vi "DAQ-AI Mean Value.vi"(11 "data":dbl[][](array[numeric]) format="%0.2f") -> (3 "Analoge Input":dbl[](array[numeric]))   [LabVIEW 2015]
uses:
  <vilib>/Analysis/baseanly.llb/Mean (DBL).vi
  Galobal variable_TI.vi
  <vilib>/Analysis/NI_AALBase.lvlib
  <vilib>/ptbypt/NI_PtbyPt.lvlib
panel:
  out "Sensor Data":T1
  out "AI_as DI":bool[](array[boolean])
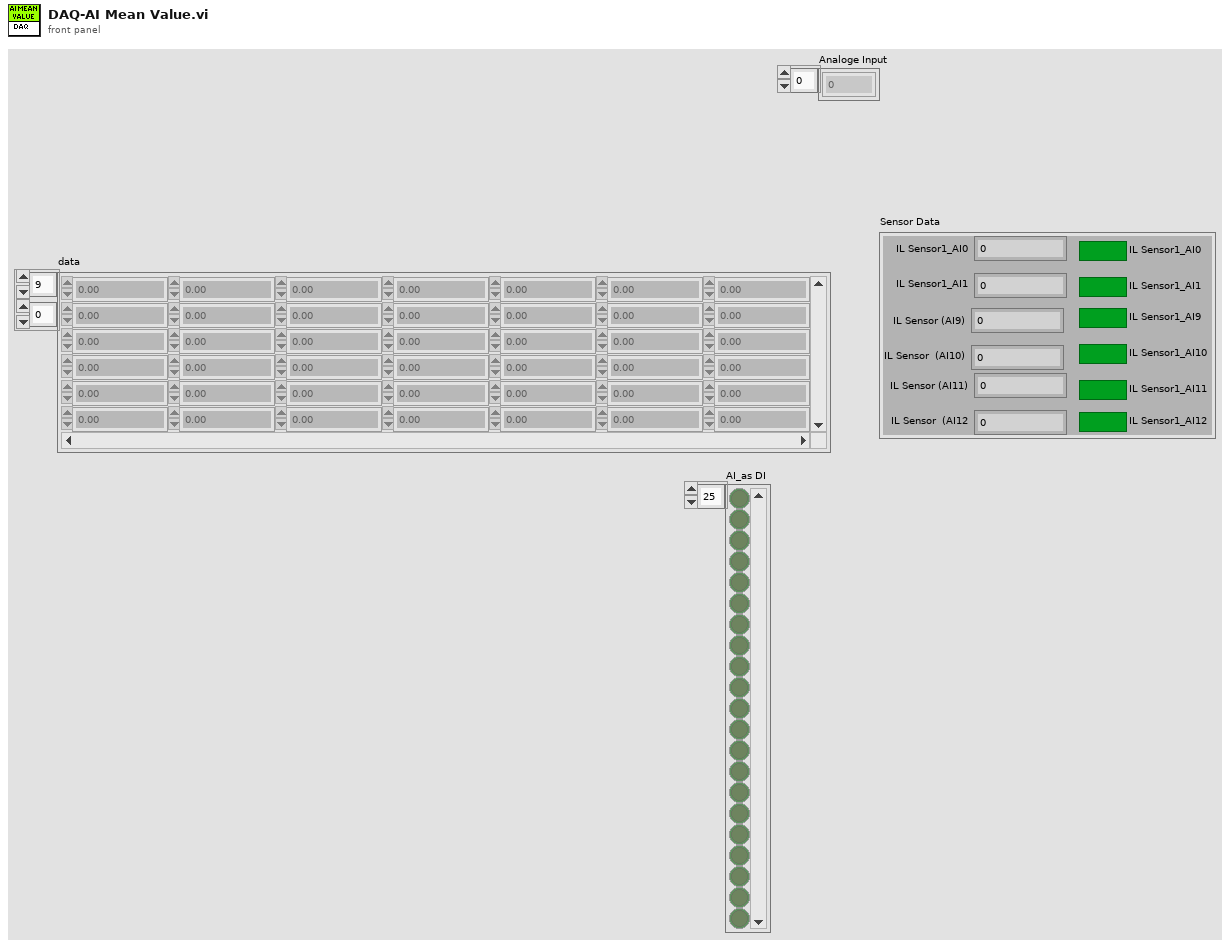
[diagram p1: front panel]
types:
  T1 = cluster{"IL Sensor1_AI0":dbl, "IL Sensor1_AI1":dbl, "IL Sensor (AI9)":dbl, "IL Sensor  (AI10)":dbl, "IL Sensor (AI11)":dbl, "IL Sensor  (AI12":dbl, "IL Sensor1_AI0":bool, "IL Sensor1_AI1":bool, "IL Sensor1_AI9":bool, "IL Sensor1_AI10":bool, "IL Sensor1_AI11":bool, "IL Sensor1_AI12":bool}
  T2 = cluster{"IL Sensor1_AI0":dbl, "IL Sensor1_AI1":dbl, "IL Sensor (AI6)":dbl, "IL Sensor  (AI7)":dbl, "IL Sensor (AI8)":dbl, "IL Sensor  (AI9)":dbl, "IL Sensor1_AI0":bool, "IL Sensor1_AI1":bool, "IL Sensor1_AI9":bool, "IL Sensor1_AI10":bool, "IL Sensor1_AI11":bool, "IL Sensor1_AI12":bool}
  T3 = cluster{"IL Sensor1_Max AI0":dbl, "IL Sensor1_Min AI0":dbl, "IL Sensor1_Max AI1":dbl, "IL Sensor1_ Min AI1":dbl, "IL Sensor_Max (AI9)":dbl, "IL Sensor_Min  (AI9)":dbl, "IL Sensor_Max (AI10)":dbl, "IL Sensor_Min(AI10)":dbl, "IL Sensor_Max (AI11)":dbl, "IL Sensor_Min (AI11)":dbl, "IL Sensor_Max (AI12)":dbl, "IL Sensor_Min (AI12":dbl}
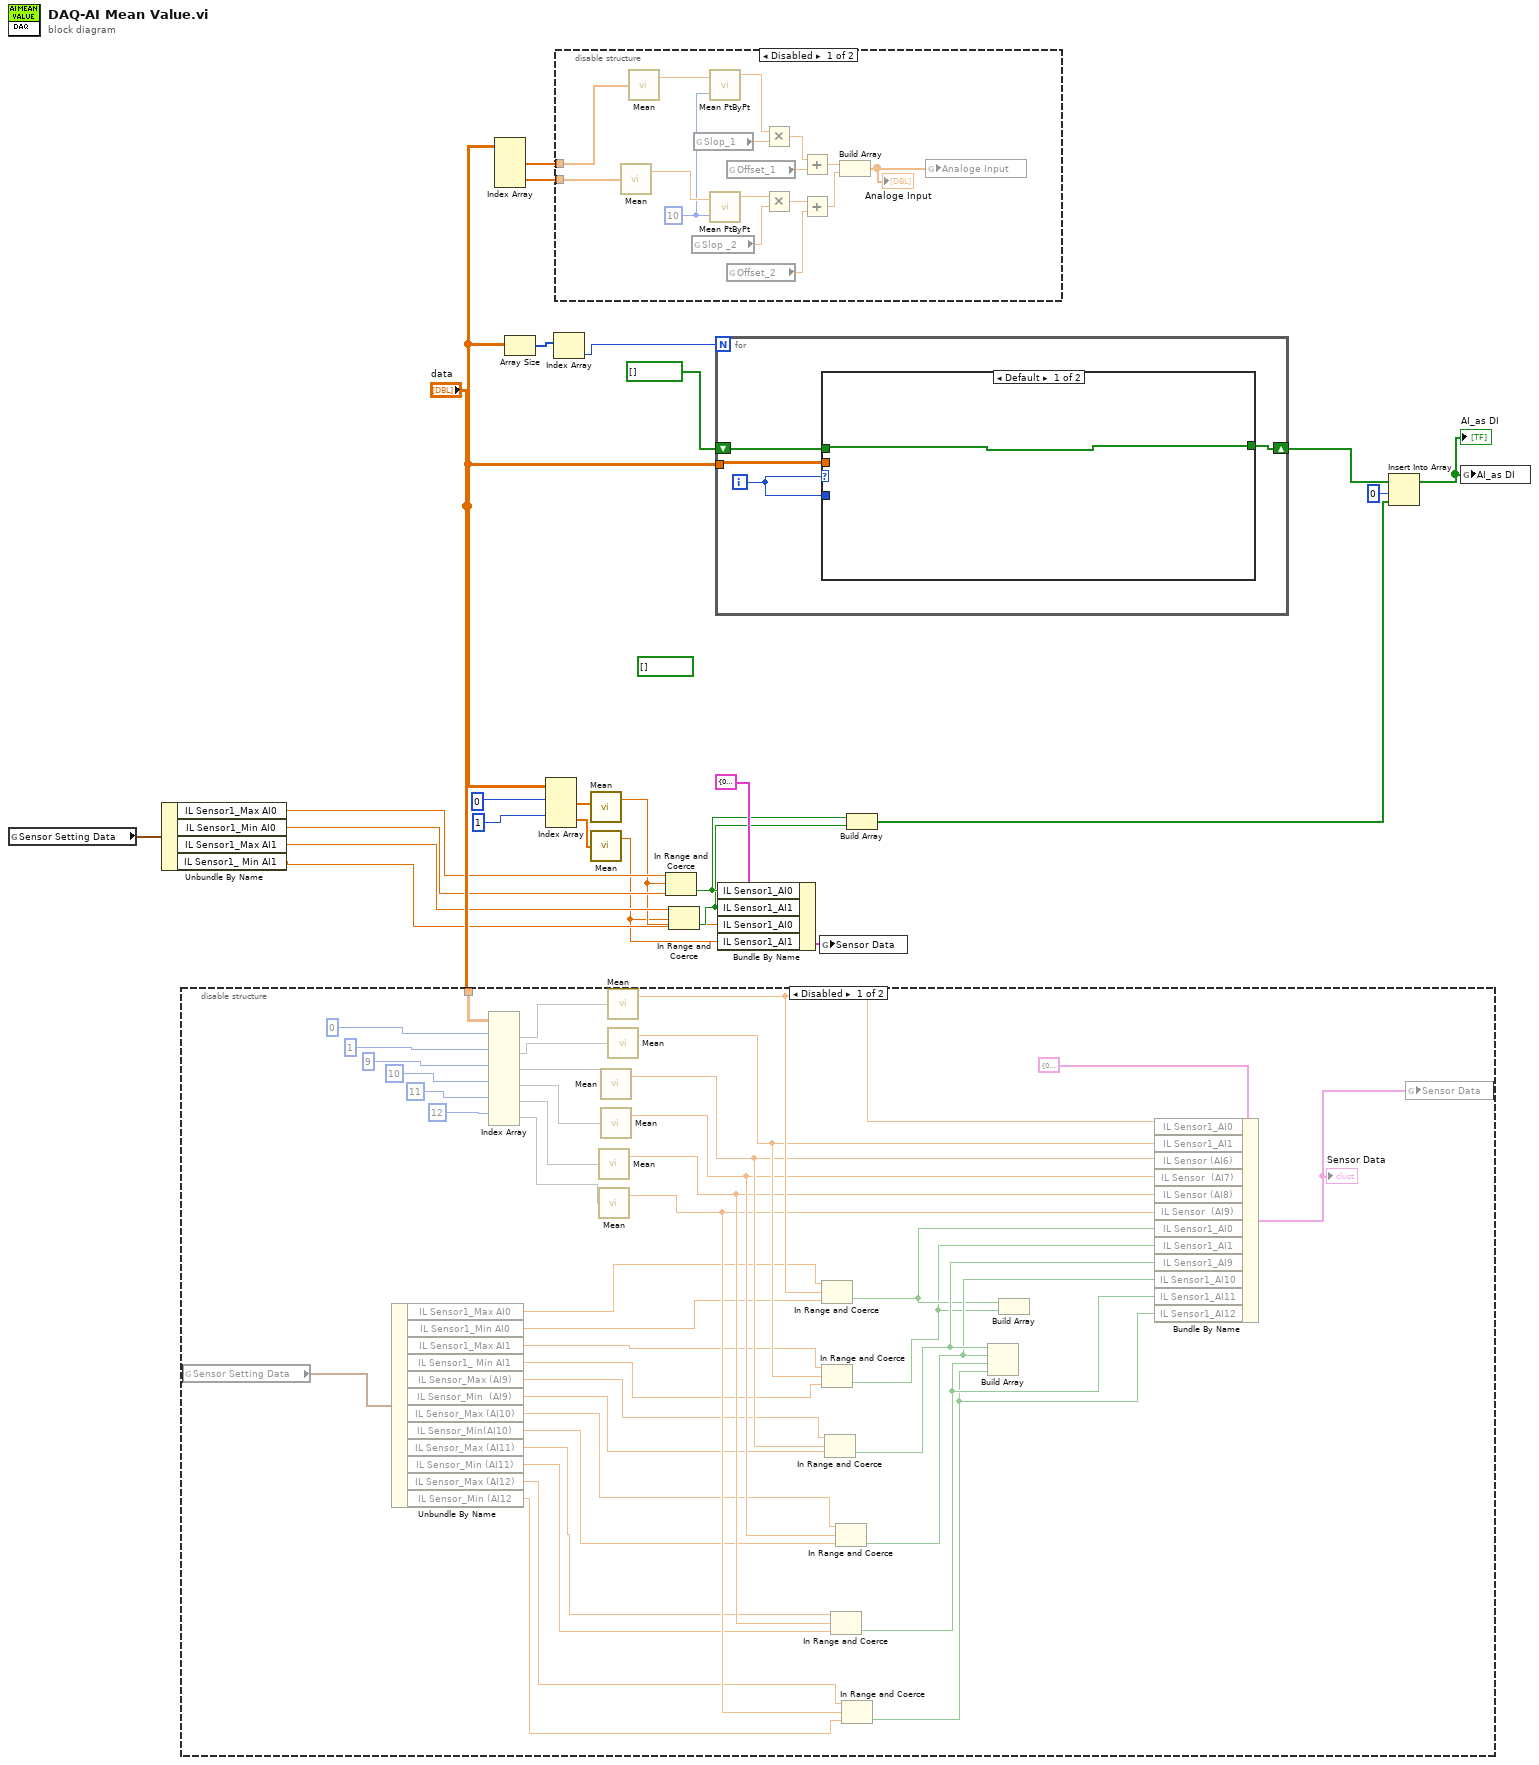
[diagram p0: block diagram]
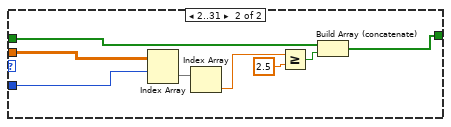
[diagram p4: hidden frame]
diagram:
  (unwired) bool[] []
  n1 = global read "Galobal variable_TI.vi" "Sensor Setting Data"() -> (w15:T3)
  n2 = Unbundle By Name(w15) -> ("IL Sensor1_Max AI0"=w14:dbl, "IL Sensor1_Min AI0"=w13:dbl, "IL Sensor1_Max AI1"=w12:dbl, "IL Sensor1_ Min AI1"=w11:dbl)
  n3 = disable-structure shown="Disabled" {
    disable-tunnel: "data" -> [w63 _]
    frame Disabled {
      n4 = global read "Galobal variable_TI.vi" "Sensor Setting Data"() -> (w26:T3)
      n5 = Unbundle By Name(w26) -> ("IL Sensor1_Max AI0"=w38:dbl, "IL Sensor1_Min AI0"=w37:dbl, "IL Sensor1_Max AI1"=w36:dbl, "IL Sensor1_ Min AI1"=w35:dbl, "IL Sensor_Max (AI9)"=w34:dbl, "IL Sensor_Min  (AI9)"=w33:dbl, "IL Sensor_Max (AI10)"=w32:dbl, "IL Sensor_Min(AI10)"=w31:dbl, "IL Sensor_Max (AI11)"=w30:dbl, "IL Sensor_Min (AI11)"=w29:dbl, "IL Sensor_Max (AI12)"=w28:dbl, "IL Sensor_Min (AI12"=w27:dbl)
      n6 = Index Array(array=w63, index (row) #1=0 ("index (row)"), index (row) #2=1 ("index (row)"), index (row) #3=9 ("index (row)"), index (row) #4=10 ("index (row)"), index (row) #5=11 ("index (row)"), index (row) #6=12 ("index (row)")) -> (element #1=w65:dbl[], element #2=w64:dbl[], element #3=w60:dbl[], element #4=w59:dbl[], element #5=w58:dbl[], element #6=w57:dbl[])  [unwired: 6 in]
      n7 = call-poly <vilib>:"Mean.vi"("X"=w58) -> ("mean"=w52:dbl)  [unwired: 1 out]
      n8 = call-poly <vilib>:"Mean.vi"("X"=w57) -> ("mean"=w51:dbl)  [unwired: 1 out]
      n9 = call-poly <vilib>:"Mean.vi"("X"=w60) -> ("mean"=w54:dbl)  [unwired: 1 out]
      n10 = call-poly <vilib>:"Mean.vi"("X"=w59) -> ("mean"=w53:dbl)  [unwired: 1 out]
      n11 = call-poly <vilib>:"Mean.vi"("X"=w65) -> ("mean"=w56:dbl)  [unwired: 1 out]
      n12 = call-poly <vilib>:"Mean.vi"("X"=w64) -> ("mean"=w55:dbl)  [unwired: 1 out]
      n13 = In Range and Coerce(upper limit=w38, x=w56, lower limit=w37) -> (In Range?=w49:bool)  [unwired: 1 out]
      n14 = In Range and Coerce(upper limit=w36, x=w55, lower limit=w35) -> (In Range?=w48:bool)  [unwired: 1 out]
      n15 = In Range and Coerce(upper limit=w34, x=w54, lower limit=w33) -> (In Range?=w62:bool)  [unwired: 1 out]
      n16 = In Range and Coerce(upper limit=w30, x=w52, lower limit=w29) -> (In Range?=w47:bool)  [unwired: 1 out]
      n17 = In Range and Coerce(upper limit=w32, x=w53, lower limit=w31) -> (In Range?=w61:bool)  [unwired: 1 out]
      n18 = In Range and Coerce(upper limit=w28, x=w51, lower limit=w27) -> (In Range?=w46:bool)  [unwired: 1 out]
      n19 = Build Array(w62, w61, w47, w46) -> ()  [unwired: 1 out]
      n20 = Build Array(w49, w48) -> ()  [unwired: 1 out]
      n21 = Bundle By Name(cluster=T2 {"IL Sensor1_AI0"=0.0, "IL Sensor1_AI1"=0.0, "IL Sensor (AI6)"=0.0, "IL Sensor  (AI7)"=0.0, "IL Sensor (AI8)"=0.0, "IL Sensor  (AI9)"=0.0, "IL Sensor1_AI0"=FALSE, "IL Sensor1_AI1"=FALSE, "IL Sensor1_AI9"=FALSE, "IL Sensor1_AI10"=FALSE, "IL Sensor1_AI11"=FALSE, "IL Sensor1_AI12"=FALSE} ("Sensor Data"), "IL Sensor1_AI0"=w56, "IL Sensor1_AI1"=w55, "IL Sensor (AI6)"=w54, "IL Sensor  (AI7)"=w53, "IL Sensor (AI8)"=w52, "IL Sensor  (AI9)"=w51, "IL Sensor1_AI0"=w49, "IL Sensor1_AI1"=w48, "IL Sensor1_AI9"=w62, "IL Sensor1_AI10"=w61, "IL Sensor1_AI11"=w47, "IL Sensor1_AI12"=w46) -> (w39:T2)
      "Sensor Data" <- w39
      n22 = global write "Galobal variable_TI.vi" "Sensor Data"(w39) -> ()
    }
    frame Enabled {
    }
  }
  n23 = Index Array(array="data") -> (element #1=w22:dbl[], element #2=w25:dbl[])  [unwired: 4 in]
  n24 = Array Size(array="data") -> (size(s)=w24:i32[])
  n25 = Index Array(array="data", index (row) #1=0 ("index (row)"), index (row) #2=1 ("index (row)")) -> (element #1=w19:dbl[], element #2=w18:dbl[])  [unwired: 2 in]
  n26 = Index Array(array=w24) -> (element=w17:i32)  [unwired: 1 in]
  n27 = disable-structure shown="Disabled" {
    disable-tunnel: w25 -> [w81 _]
    disable-tunnel: w22 -> [w78 _]
    frame Disabled {
      w77 = 10 ("sample length")
      n28 = call-poly <vilib>:"Mean.vi"("X"=w81) -> ("mean"=w79:dbl)  [unwired: 1 out]
      n29 = call-poly <vilib>:"Mean.vi"("X"=w78) -> ("mean"=w80:dbl)  [unwired: 1 out]
      n30 = global read "Galobal variable_TI.vi" "Slop _2"() -> (w69:dbl)
      n31 = global read "Galobal variable_TI.vi" "Slop_1"() -> (w74:dbl)
      n32 = call <vilib>:"Mean PtByPt.vi"("x"=w80, "sample length"=w77) -> ("mean"=w75:dbl)  [unwired: 2 in, 1 out]
      n33 = call <vilib>:"Mean PtByPt.vi"("x"=w79, "sample length"=w77) -> ("mean"=w70:dbl)  [unwired: 2 in, 1 out]
      n34 = global read "Galobal variable_TI.vi" "Offset_1"() -> (w72:dbl)
      n35 = global read "Galobal variable_TI.vi" "Offset_2"() -> (w68:dbl)
      n36 = Multiply(x=w75, y=w74) -> (x*y=w73:dbl)
      n37 = Multiply(x=w70, y=w69) -> (x*y=w71:dbl)
      n38 = Add(x=w73, y=w72) -> (x+y=w67:dbl)
      n39 = Add(x=w71, y=w68) -> (x+y=w66:dbl)
      n40 = Build Array(w67, w66) -> (w76:dbl[])
      "Analoge Input" <- w76
      n41 = global write "Galobal variable_TI.vi" "Analoge Input"(w76) -> ()
    }
    frame Enabled {
    }
  }
  n42 = call-poly <vilib>:"Mean.vi"("X"=w19) -> ("mean"=w2:dbl)  [unwired: 1 out]
  n43 = call-poly <vilib>:"Mean.vi"("X"=w18) -> ("mean"=w1:dbl)  [unwired: 1 out]
  n44 = In Range and Coerce(upper limit=w14, x=w2, lower limit=w13) -> (In Range?=w7:bool)  [unwired: 1 out]
  n45 = In Range and Coerce(upper limit=w12, x=w1, lower limit=w11) -> (In Range?=w6:bool)  [unwired: 1 out]
  n46 = for {
    N: w17 -> [_]
    tunnel: "data" -> [w85]
    shift-right: [w82] -> w8
    shift-left: bool[] [] -> [w83]
    i -> [w84]
    n47 = case shown="Default" w84 {
      tunnel: w85 -> [_ w94]
      tunnel: w84 -> [_ w92]
      tunnel: [w86 w87] -> w82
      tunnel: w83 -> [w86 w93]
      frame Default {
      }
      frame 2..31 {
        n48 = Index Array(array=w94, index (row)=w92) -> (element=w89:dbl[])  [unwired: 1 in]
        n49 = Index Array(array=w89) -> (element=w91:dbl)  [unwired: 1 in]
        n50 = Greater Or Equal?(x=w91, y=2.5) -> (x >= y?=w88:bool)
        n51 = Build Array (concatenate)(w93, w88) -> (w87:bool[])
      }
    }
  }
  n52 = Bundle By Name(cluster=T2 {"IL Sensor1_AI0"=0.0, "IL Sensor1_AI1"=0.0, "IL Sensor (AI6)"=0.0, "IL Sensor  (AI7)"=0.0, "IL Sensor (AI8)"=0.0, "IL Sensor  (AI9)"=0.0, "IL Sensor1_AI0"=FALSE, "IL Sensor1_AI1"=FALSE, "IL Sensor1_AI9"=FALSE, "IL Sensor1_AI10"=FALSE, "IL Sensor1_AI11"=FALSE, "IL Sensor1_AI12"=FALSE} ("Sensor Data"), "IL Sensor1_AI0"=w7, "IL Sensor1_AI1"=w6, "IL Sensor1_AI0"=w2, "IL Sensor1_AI1"=w1) -> (w9:T2)
  n53 = global write "Galobal variable_TI.vi" "Sensor Data"(w9) -> ()
  n54 = Build Array(w7, w6) -> (w5:bool[])
  n55 = Insert Into Array(array=w8, index=0, new element=w5) -> (w3:bool[])
  "AI_as DI" <- w3
  n56 = global write "Galobal variable_TI.vi" "AI_as DI"(w3) -> ()
